vi "solar Create (LVClass).vi"(8 "error in (no error)":errorcluster, 10 "LVClass (*.lvclass)":string, 11 "Default LVClass":refnum<class "solar.lvclass">) -> (0 "error out":errorcluster, 2 "dup Default LVClass":refnum<class "solar.lvclass">, 3 "solar out":refnum<class "solar.lvclass">)   [LabVIEW 2018, in "solar.lvclass"]
doc: "This loads a target's LabVIEW Class from memory. Target inheritance expands the default functionality of a SOLAR target."
uses:
  solar.lvclass
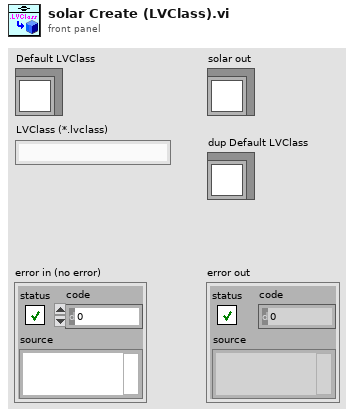
[diagram p1: front panel]
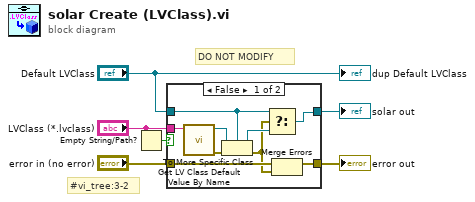
[diagram p0: block diagram]
diagram:
  # "#vi_tree:3-2"
  # "DO NOT MODIFY"
  n1 = Empty String/Path?(string/path="LVClass (*.lvclass)") -> (empty?=w6:bool)
  n2 = case shown="False" w6 {
    tunnel: [w11 w17] -> w2
    tunnel: "Default LVClass" -> [w12 w17]
    tunnel: [w9 w16] -> w1
    tunnel: "error in (no error)" -> [w10 w16]
    tunnel: "LVClass (*.lvclass)" -> [w7 _]
    frame False {
      n3 = call <vilib>:"Get LV Class Default Value By Name.vi"("class name"=w7) -> ("error out"=w15:errorcluster, "object"=w14:refnum<class>)  [unwired: 9 in]
      n4 = To More Specific Class(target class=w12, reference=w14, error in=w15) -> (specific class reference=w13:refnum<class "solar.lvclass">, error out=w8:errorcluster)
      n5 = Select(t=w12, s=w8, f=w13) -> (s? t:f=w11:refnum<class "solar.lvclass">)
      n6 = Merge Errors(w10, w8) -> (w9:errorcluster)
    }
    frame True {
    }
  }
  "error out" <- w1
  "solar out" <- w2
  "dup Default LVClass" <- "Default LVClass"
